vi "Stream.vi"(8 "error in":errorcluster, 11 "Node Ptr":T2 format="%.0x") -> (0 "error out":errorcluster)   [LabVIEW 2026, in "Nominal Core Streaming System Explorer.lvlib"]
uses:
  Nominal Core Streaming System Explorer.lvlib
  <vilib>/NI VeriStand/Custom Device API/Custom Device Item Ref.ctl
  Shared/stream configuration mode.ctl
  Shared/Constants.vi
  <vilib>/NI VeriStand/Custom Device API/Custom Device API.lvlib
  Shared/Nominal Core Streaming Shared.lvlib
  <vilib>/NI VeriStand/Custom Device Tools/Custom Device Utility Library/Custom Device Utility Library.lvlib
panel:
  in  "Remove":bool
  in  "Add Channels":bool
  in  "Logged Channels":i32[](listbox)
  in  "Dataset RID":string
  in  "identifier selection":T1
  in  "Dataset Name":string
  in  "Asset RID":string
  in  "Description":string
  in  "Name":string
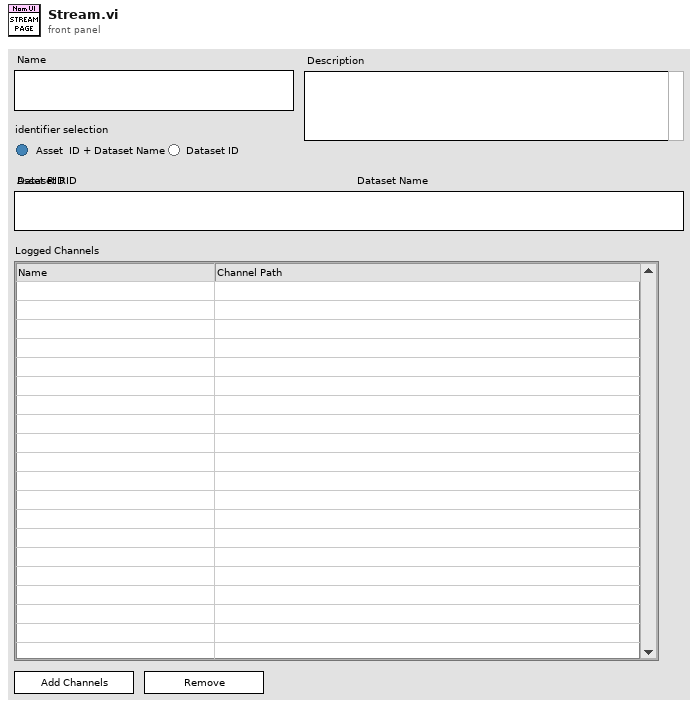
[diagram p1: front panel]
types:
  T1 = typedef "Nominal Core Streaming Shared.lvlib/stream configuration mode.ctl" = enum32{"asset+dsname", "dsetid"}
  T2 = typedef "Custom Device API.lvlib/Custom Device Item Ref.ctl" = u64
  T3 = typedef "Custom Device API.lvlib/Custom Device Item Info.ctl" = cluster{"Name":string, "Is Channel":bool, "GUID":string, "Is Waveform":bool}
  T4 = typedef "Custom Device API.lvlib/Custom Device Commands.ctl" = enum16{"Default", "Item renamed", "Shutdown", "Dynamic button pressed"}
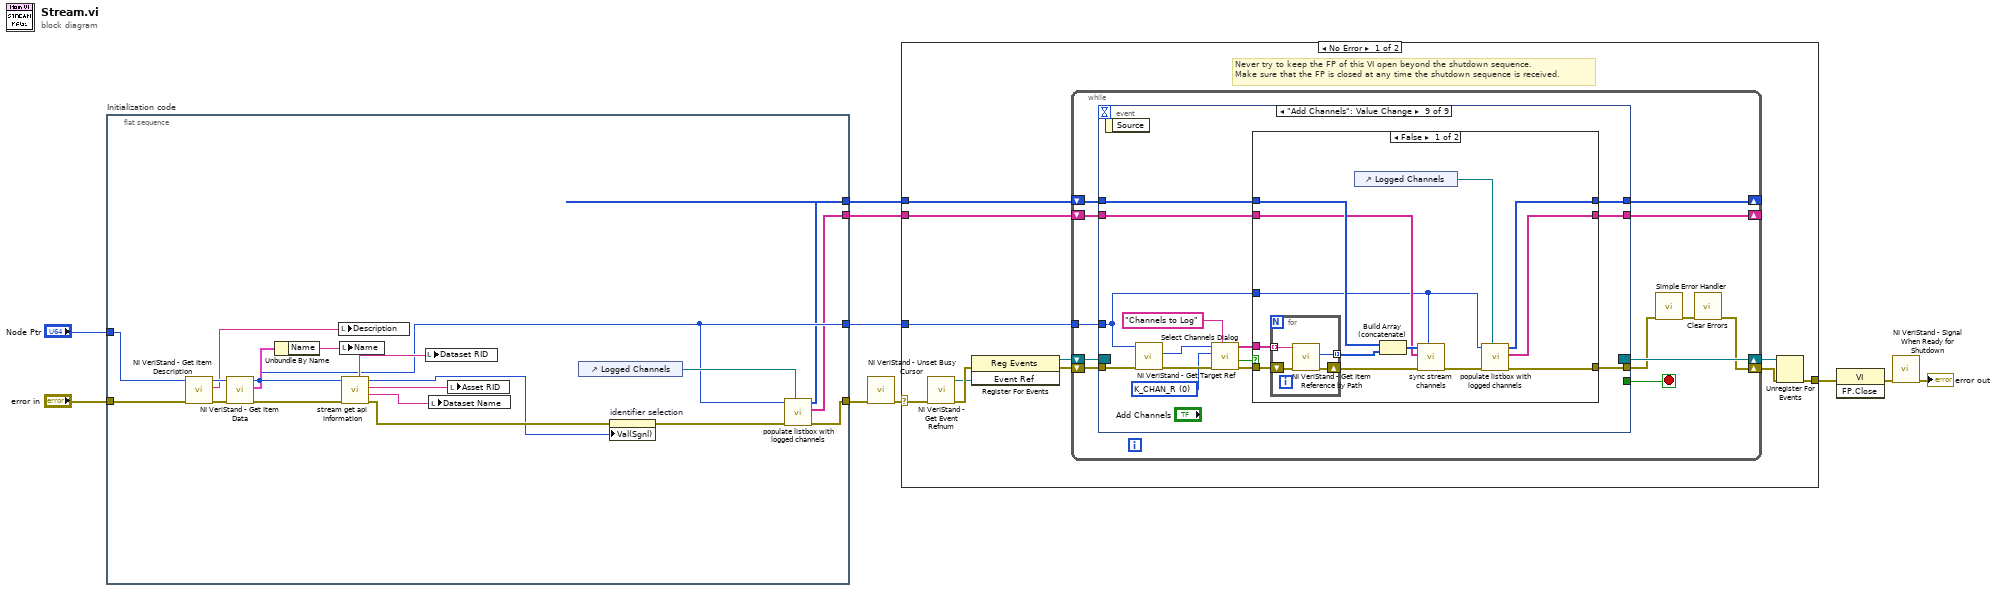
[diagram p0: block diagram]
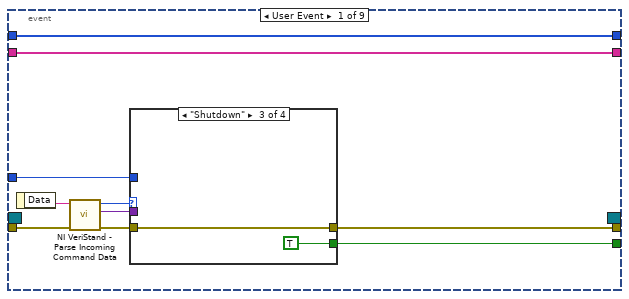
[diagram p2: hidden frame]
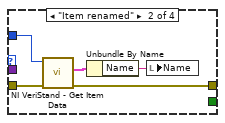
[diagram p4: hidden frame]
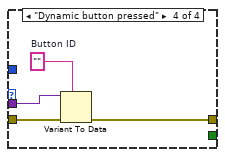
[diagram p5: hidden frame]
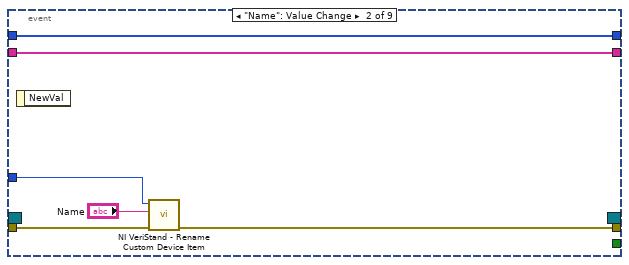
[diagram p6: hidden frame]
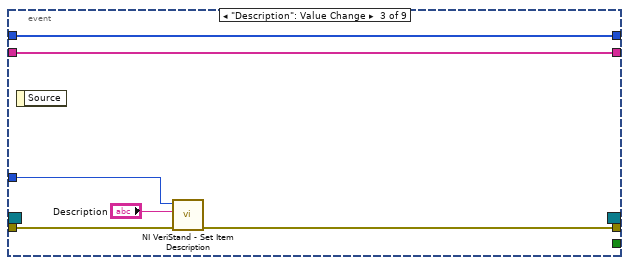
[diagram p7: hidden frame]
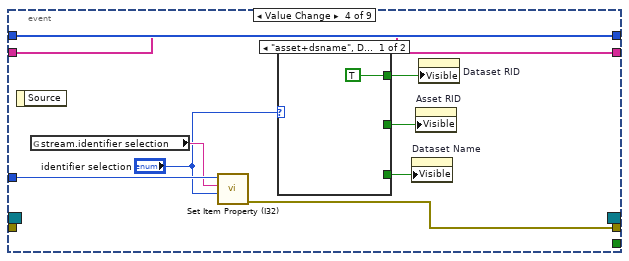
[diagram p8: hidden frame]
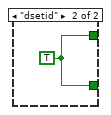
[diagram p9: hidden frame]
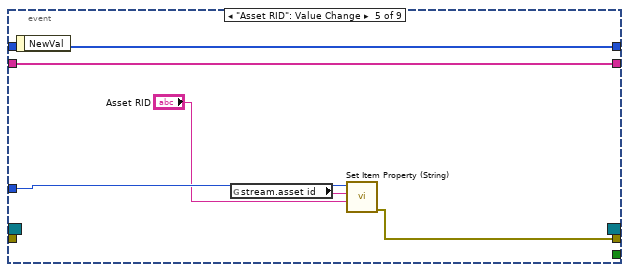
[diagram p10: hidden frame]
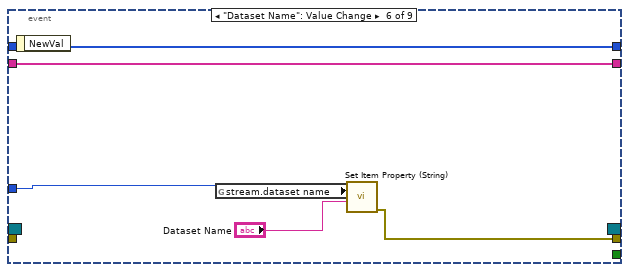
[diagram p11: hidden frame]
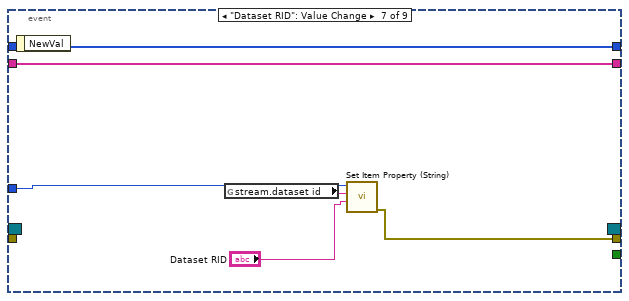
[diagram p12: hidden frame]
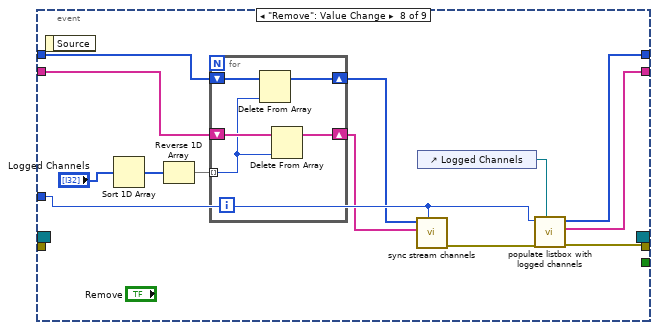
[diagram p13: hidden frame]
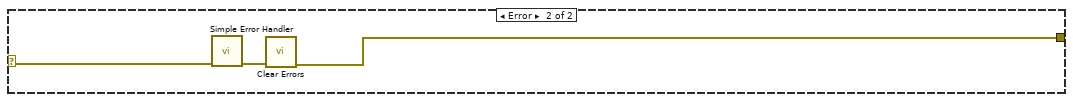
[diagram p15: hidden frame]
diagram:
  n1 = flat-sequence "Initialization code" {
    tunnel: "error in" -> [w22]
    tunnel: "Node Ptr" -> [w25]
    tunnel: [w17] -> w6
    tunnel: [w14] -> w3
    tunnel: [w13] -> w2
    tunnel: [w12] -> w1
    frame #0 {
      n2 = call <vilib>:"NI VeriStand - Get Item Description.vi"("error in (no error)"=w22, "Item Ref in"=w25) -> ("error out"=w28:errorcluster, "Description"=w23:string, "Item Ref out"=w29:T2)  [unwired: 7 out]
      n3 = call <vilib>:"NI VeriStand - Get Item Data.vi"("error in (no error)"=w28, "Item Ref in"=w29) -> ("error out"=w26:errorcluster, "Item Info"=w27:T3, "Item Ref out"=w14:T2)  [unwired: 7 out]
      n4 = Unbundle By Name(w27) -> ("Name"=w24:string)
      n5 = local write "Description"(w23) -> ()
      n6 = local write "Name"(w24) -> ()
      n7 = call "stream get api information.vi"("error in"=w26, "stream in"=w14) -> ("error out"=w18:errorcluster, "asset ID"=w21:string, "dataset name"=w20:string, "ID selection"=w11:T1, "dataset ID"=w19:string)  [unwired: 5 in]
      n8 = local write "Dataset RID"(w19) -> ()
      n9 = local write "Dataset Name"(w21) -> ()
      n10 = local write "Asset RID"(w20) -> ()
      n11 = control-ref of="Logged Channels"() -> (w15:refnum<vi>)
      n12 = property on="identifier selection" class="RadioBtnsControl (strict)"(error in=w18, "Val(Sgnl)"=w11) -> (error out=w16:errorcluster)  [unwired: 1 in, 1 out]
      n13 = call "populate listbox with logged channels.vi"("MulticolumnListbox in"=w15, "error in"=w16, "Item Ref in"=w14) -> ("error out"=w17:errorcluster, "logged channel shortnames"=w12:string[], "logged channel refs"=w13:T2[])  [unwired: 6 in]
    }
  }
  n14 = call <vilib>:"NI VeriStand - Unset Busy Cursor.vi"("error in (no error)"=w6) -> ("error out"=w5:errorcluster)  [unwired: 10 out]
  n15 = case shown="No Error" w5 {
    selector: w5 -> [w32 w170]
    tunnel: [w37 w168] -> w10
    tunnel: w3 -> [w33 _]
    tunnel: w2 -> [w31 _]
    tunnel: w1 -> [w30 _]
    frame No Error {
      # "Never try to keep the FP of this VI open beyond the shutdown sequence.\nMake sure that the FP is closed at any time the shutdown sequence is received."
      n16 = call <vilib>:"NI VeriStand - Get Event Refnum.vi"("error in (no error)"=w32) -> ("error out"=w40:errorcluster, "Event Ref"=w36:refnum<user-event>)  [unwired: 9 out]
      n17 = register-events(error in=w40, w36) -> (reference out=w34:refnum<event-registration>, error out=w35:errorcluster)  [unwired: 1 in]
      n18 = while {
        tunnel: w33 -> [w48]
        shift-right: [w45] -> w38
        shift-left: w35 -> [w51]
        shift-right: [w52] -> w39
        shift-left: w34 -> [w50]
        shift-right: [w42] -> _
        shift-left: w31 -> [w44]
        shift-right: [w41] -> _
        shift-left: w30 -> [w43]
        stop <- w49 stop-if-true
        n19 = event shown="[8] \"Add Channels\": Value Change" {
          selector: w50 -> [_ _ _ _ _ _ _ _ _]
          dyn-events: [_ _ _ _ _ _ _ _ _] -> w52
          timeout: _ -> [_ _ _ _ _ _ _ _ _]
          tunnel: w51 -> [w62 w80 w85 _ _ _ _ _ w147]
          tunnel: [w58 _ _ _ _ _ _ _ _] -> w49
          tunnel: [w57 w79 w84 w94 w100 w107 w113 w128 w137] -> w47
          tunnel: w48 -> [w56 w78 w86 w95 w103 w109 w115 w123 w134]
          tunnel: w44 -> [w54 w76 w82 w88 w99 w105 w111 w119 w140]
          tunnel: w43 -> [w53 w75 w81 w87 w98 w104 w110 w117 w139]
          tunnel: [w54 w76 w82 w88 w99 w105 w111 w127 w141] -> w42
          tunnel: [w53 w75 w81 w87 w98 w104 w110 w126 w138] -> w41
          event User Event {
            n20 = event-data() -> ("Data"=w61:string)  [unwired: 1 out]
            n21 = call <vilib>:"NI VeriStand - Parse Incoming Command Data.vi"("error in (no error)"=w62, "Incoming data"=w61) -> ("error out"=w60:errorcluster, "Outgoing data"=w55:variant, "Action"=w59:T4)  [unwired: 7 out]
            n22 = case shown="\"Shutdown\"" w59 {
              tunnel: w60 -> [w63 w68 w69 w74]
              tunnel: [_ _ TRUE _] -> w58
              tunnel: [w63 w65 w69 w71] -> w57
              tunnel: w56 -> [_ w67 _ _]
              tunnel: w55 -> [_ _ _ w73]
              frame "Default", Default {
              }
              frame "Item renamed" {
                n23 = call <vilib>:"NI VeriStand - Get Item Data.vi"("error in (no error)"=w68, "Item Ref in"=w67) -> ("error out"=w65:errorcluster, "Item Info"=w66:T3)  [unwired: 8 out]
                n24 = Unbundle By Name(w66) -> ("Name"=w64:string)
                n25 = local write "Name"(w64) -> ()
              }
              frame "Shutdown" {
              }
              frame "Dynamic button pressed" {
                w72 = ""  # Button ID
                n26 = Variant To Data(error in=w74, type=w72, Variant=w73) -> (error out=w71:errorcluster)  [unwired: 1 out]
              }
            }
          }
          event "Name": Value Change {
            n27 = event-data() -> ()  [unwired: 2 out]
            n28 = call <vilib>:"NI VeriStand - Rename Custom Device Item.vi"("error in (no error)"=w80, "New Name"="Name", "Item Ref in"=w78) -> ("error out"=w79:errorcluster)  [unwired: 1 in, 7 out]
          }
          event "Description": Value Change {
            n29 = event-data() -> ()  [unwired: 2 out]
            n30 = call <vilib>:"NI VeriStand - Set Item Description.vi"("error in (no error)"=w85, "Description"="Description", "Item Ref in"=w86) -> ("error out"=w84:errorcluster)  [unwired: 8 out]
          }
          event Value Change {
            n31 = event-data() -> ()  [unwired: 2 out]
            n32 = global read "Constants.vi" "stream.identifier selection"() -> (w93:string)
            n33 = call <vilib>:"Set Item Property (I32).vi"("Value"="identifier selection", "Property Name"=w93, "Item Ref in"=w95) -> ("error out"=w94:errorcluster)  [unwired: 6 in, 2 out]
            n34 = case shown="\"asset+dsname\", Default" "identifier selection" {
              tunnel: [_ w97] -> w92
              tunnel: [_ w97] -> w91
              tunnel: [TRUE _] -> w90
              frame "asset+dsname", Default {
              }
              frame "dsetid" {
                w97 = TRUE
              }
            }
            n35 = property on="Dataset Name" class="Str"("Visible"=w92) -> ()  [unwired: 2 in, 2 out]
            n36 = property on="Asset RID" class="Str"("Visible"=w91) -> ()  [unwired: 2 in, 2 out]
            n37 = property on="Dataset RID" class="Str"("Visible"=w90) -> ()  [unwired: 2 in, 2 out]
          }
          event "Asset RID": Value Change {
            n38 = event-data() -> ()  [unwired: 2 out]
            n39 = global read "Constants.vi" "stream.asset id"() -> (w101:string)
            n40 = call <vilib>:"Set Item Property (String).vi"("Value"="Asset RID", "Property Name"=w101, "Item Ref in"=w103) -> ("error out"=w100:errorcluster)  [unwired: 6 in, 2 out]
          }
          event "Dataset Name": Value Change {
            n41 = event-data() -> ()  [unwired: 2 out]
            n42 = global read "Constants.vi" "stream.dataset name"() -> (w108:string)
            n43 = call <vilib>:"Set Item Property (String).vi"("Value"="Dataset Name", "Property Name"=w108, "Item Ref in"=w109) -> ("error out"=w107:errorcluster)  [unwired: 6 in, 2 out]
          }
          event "Dataset RID": Value Change {
            n44 = event-data() -> ()  [unwired: 2 out]
            n45 = global read "Constants.vi" "stream.dataset id"() -> (w114:string)
            n46 = call <vilib>:"Set Item Property (String).vi"("Value"="Dataset RID", "Property Name"=w114, "Item Ref in"=w115) -> ("error out"=w113:errorcluster)  [unwired: 6 in, 2 out]
          }
          event "Remove": Value Change {
            n47 = event-data() -> ()  [unwired: 2 out]
            n48 = Sort 1D Array(array="Logged Channels") -> (sorted array=w122:i32[])
            n49 = Reverse 1D Array(array=w122) -> (reversed array=w120:i32[])
            n50 = for {
              tunnel: w120 -> [w129] mode=indexing
              shift-right: [w132] -> w118
              shift-left: w119 -> [w133]
              shift-right: [w130] -> w116
              shift-left: w117 -> [w131]
              n51 = Delete From Array(array=w133, index=w129) -> (array with subset deleted=w132:T2[])  [unwired: 1 in, 1 out]
              n52 = Delete From Array(array=w131, index=w129) -> (array with subset deleted=w130:string[])  [unwired: 1 in, 1 out]
            }
            n53 = call "sync stream channels.vi"("stream"=w123, "names"=w116, "channels"=w118) -> ("error out"=w124:errorcluster)  [unwired: 6 in, 2 out]
            n54 = control-ref of="Logged Channels"() -> (w125:refnum<vi>)
            n55 = call "populate listbox with logged channels.vi"("MulticolumnListbox in"=w125, "error in"=w124, "Item Ref in"=w123) -> ("error out"=w128:errorcluster, "logged channel shortnames"=w126:string[], "logged channel refs"=w127:T2[])  [unwired: 6 in]
          }
          event "Add Channels": Value Change {
            w143 = u8 0 items=["K_CHAN_R", "K_CHAN_W", "K_CHAN_RW", "K_CHAN_VOLT", "K_CHAN_FAULT", "K_ALL", "K_CUSTOM"] ("Filter")
            n56 = event-data() -> ()  [unwired: 2 out]
            n57 = call <vilib>:"NI VeriStand - Get Target Ref.vi"("error in"=w147, "Item Ref in"=w134) -> ("error out"=w145:errorcluster, "Target Ref"=w146:T2)  [unwired: 6 in, 2 out]
            n58 = call "Select Channels Dialog.vi"("Tree header"="Channels to Log", "error in (no error)"=w145, "Filter"=w143, "Start Item Ref"=w146) -> ("error out"=w136:errorcluster, "Canceled"=w142:bool, "Channel paths"=w135:string[])  [unwired: 5 in]
            n59 = case shown="False" w142 {
              tunnel: [w150 w167] -> w141
              tunnel: w140 -> [w156 w167]
              tunnel: w139 -> [w154 w166]
              tunnel: [w149 w166] -> w138
              tunnel: [w148 w165] -> w137
              tunnel: w136 -> [w159 w165]
              tunnel: w135 -> [w160 _]
              tunnel: w134 -> [w152 _]
              frame False {
                n60 = for {
                  shift-right: [w163] -> w158
                  shift-left: w159 -> [w164]
                  tunnel: w160 -> [w162] mode=indexing
                  tunnel: [w161] -> w157 mode=indexing
                  n61 = call <vilib>:"NI VeriStand - Get Item Reference by Path.vi"("error in (no error)"=w164, "Item Path in"=w162) -> ("error out"=w163:errorcluster, "Item Ref"=w161:T2)  [unwired: 6 in, 2 out]
                }
                n62 = control-ref of="Logged Channels"() -> (w151:refnum<vi>)
                n63 = Build Array (concatenate)(w156, w157) -> (w155:T2[])
                n64 = call "sync stream channels.vi"("stream"=w152, "error in"=w158, "names"=w154, "channels"=w155) -> ("error out"=w153:errorcluster)  [unwired: 5 in, 2 out]
                n65 = call "populate listbox with logged channels.vi"("MulticolumnListbox in"=w151, "error in"=w153, "Item Ref in"=w152) -> ("error out"=w148:errorcluster, "logged channel shortnames"=w149:string[], "logged channel refs"=w150:T2[])  [unwired: 6 in]
              }
              frame True {
              }
            }
          }
        }
        n66 = call <vilib>:"Simple Error Handler.vi"("error in (no error)"=w47) -> ("error out"=w46:errorcluster)  [unwired: 1 in, 7 out]
        n67 = call <vilib>:"Clear Errors.vi"("error in (no error)"=w46) -> ("error out"=w45:errorcluster)  [unwired: 1 in, 5 out]
      }
      n68 = Unregister For Events(event registration refnum=w39, error in=w38) -> (error out=w37:errorcluster)
    }
    frame Error {
      n69 = call <vilib>:"Simple Error Handler.vi"("error in (no error)"=w170) -> ("error out"=w169:errorcluster)  [unwired: 1 in, 7 out]
      n70 = call <vilib>:"Clear Errors.vi"("error in (no error)"=w169) -> ("error out"=w168:errorcluster)  [unwired: 1 in, 5 out]
    }
  }
  n71 = invoke class="VI" method="FP.Close"(error in=w10) -> (error out=w9:errorcluster)  [unwired: 2 in, 2 out]
  n72 = call <vilib>:"NI VeriStand - Signal When Ready for Shutdown.vi"("error in (no error)"=w9) -> ("error out"=→"error out":errorcluster)  [unwired: 10 out]
